vi "Read Details.vi"(11 "Protected Actor Handle in":refnum<class "Protected Actor Handle.lvclass">) -> (2 "Actor Details":T1)   [LabVIEW 2020, in "AF Debug.lvlib" / "Protected Actor Handle.lvclass"]
doc: "Reads identification information about the actor, useful for display in a debugger."
uses:
  Protected Actor Handle.lvclass
  Protected Actor Handle.lvclass/Protected Actor Handle.ctl
  vi.lib/ActorFramework/Inspection API/Protected Actor Handle/Protected Actor Handle.lvclass
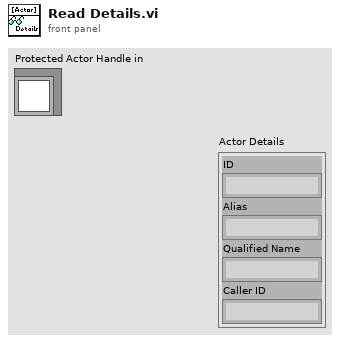
[diagram p1: front panel]
types:
  T1 = cluster{"ID":string, "Alias":string, "Qualified Name":string, "Caller ID":string}
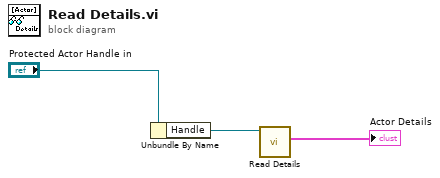
[diagram p0: block diagram]
diagram:
  n1 = Unbundle By Name("Protected Actor Handle in") -> ("Handle"=w2:refnum<class "Protected Actor Handle.lvclass">)
  n2 = call "Read Details.vi"("Protected Actor Handle in"=w2) -> ("Actor Details"=→"Actor Details":T1)  [unwired: 10 in]
